vi "3Dpathlength.vi"(6 "Exclude Array":T1[](array[typedef])=[{"Sizes"=[{"Max"=15000.0, "Min"=0.0}, {"Max"=1000.0, "Min"=-1000.0}, {"Max"=300.0, "Min"=0.0}], "Name"="Roughness Elements", "Exclude Type"=enum."Allow only vertical moves"}, {"Sizes"=[{"Max"=17000.0, "Min"=16000.0}, {"Max"=200.0, "Min"=-200.0}, {"Max"=-50.0, "Min"=-250.0}], "Name"="B204", "Exclude Type"=enum."Exclude completely"}] {"Sizes"."Min" format="%#.1f"; "Sizes"."Max" format="%#.1f"}, 11 "targetCoords":sgl[][](array[numeric])) -> (1 "Zs":sgl[](array[numeric]), 2 "Ys":sgl[](array[numeric]), 3 "Xs":sgl[](array[numeric]), 4 "pathlength":sgl)   [LabVIEW 2021]
uses:
  Gen Trav/Route mapping/Box_size.ctl
  Gen Trav/Route mapping/Exclusion_type.ctl
  Gen Trav/Route mapping/Exclude_cluster.ctl
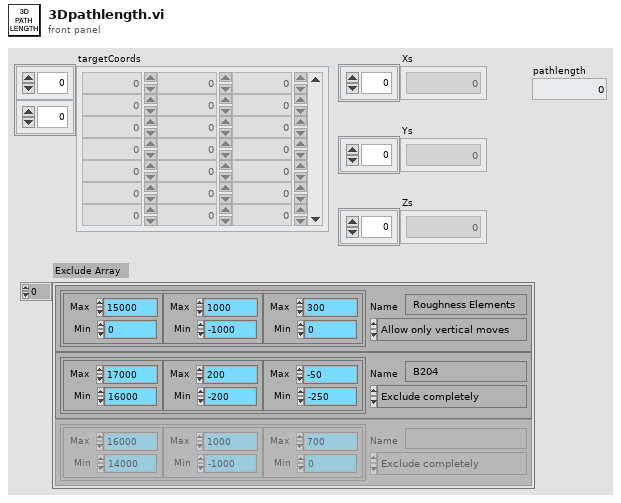
[diagram p1: front panel]
types:
  T1 = typedef "Exclude_cluster.ctl" = cluster{"Sizes":T2, "Name":string, "Exclude Type":T3}
  T2 = typedef "Box_size.ctl" = cluster{"Max":sgl, "Min":sgl}[]
  T3 = typedef "Exclusion_type.ctl" = enum16{"Exclude completely", "Allow only vertical moves"}
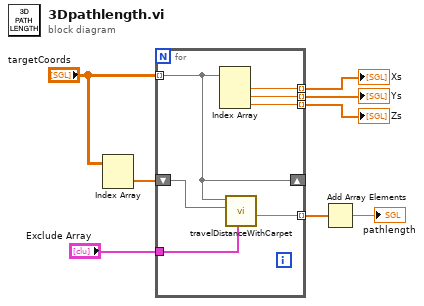
[diagram p0: block diagram]
diagram:
  n1 = Index Array(array="targetCoords") -> (element=w2:sgl[])  [unwired: 2 in]
  n2 = for {
    tunnel: [w15] -> w8 mode=indexing
    tunnel: [w14] -> w7 mode=indexing
    tunnel: [w13] -> w6 mode=indexing
    shift-right: [w12] -> _
    shift-left: w2 -> [w11]
    tunnel: [w10] -> w5 mode=indexing
    tunnel: "targetCoords" -> [w12] mode=indexing
    tunnel: "Exclude Array" -> [w9]
    n3 = Index Array(array=w12) -> (element #1=w15:sgl, element #2=w14:sgl, element #3=w13:sgl)  [unwired: 3 in]
    n4 = call "travelDistanceWithCarpet.vi"("Exclude Array"=w9, "pointB"=w11, "pointA"=w12) -> ("distance"=w10:dbl)  [unwired: 7 in, 1 out]
  }
  "Xs" <- w8
  "Ys" <- w7
  "Zs" <- w6
  n5 = Add Array Elements(numeric array=w5) -> (sum=→"pathlength":dbl)
